vi "Test UI-Bus Boolean Vars.vi"() -> ()   [LabVIEW 2021]
uses:
  Source/UI-Bus/UI-Bus.lvclass
  C:/Program Files (x86)/National Instruments/LabVIEW 2021/vi.lib/TSA/Omni-Bus/Omni-Bus/Bus Access/Bus_Access.lvclass
  <vilib>/TSA/Omni-Bus/Omni-Bus/Omni_Bus.lvclass
  <vilib>/TSA/Omni-Bus/Omni-Bus/Support/Broad Types.ctl
  <vilib>/TSA/Abstract Data Classes/Abs_Types/Type/Abs_Type.lvclass/Abs_Type.ctl
  <vilib>/TSA/Omni-Bus/Omni-Bus/Omni_Bus.lvclass/Omni_Bus.ctl
  <vilib>/TSA/Omni-Bus/Omni-Bus/Support/Read/Read Multi Boolean.vi
  <vilib>/TSA/Omni-Bus/Omni-Bus/Support/Write/Write Boolean.vi
  <vilib>/TSA/Omni-Bus/Omni-Bus/Support/Get/Get Multi Boolean.vi
  <vilib>/TSA/Omni-Bus/Omni-Bus/Support/FindVar.vi
  <vilib>/TSA/Omni-Bus/Omni-Bus/Support/FindMultiVar.vi
  <vilib>/Utility/error.llb/Clear Errors.vi
  <vilib>/TSA/Omni-Bus/Omni-Bus/Properties/Read Var Map.vi
  <vilib>/TSA/Abstract Data Classes/Abs_Types/Type/Properties/Read Tag.vi
  <vilib>/TSA/Abstract Data Classes/Abs_Types/Boolean/Abs_Boolean.lvclass
  C:/Program Files (x86)/National Instruments/LabVIEW 2021/vi.lib/TSA/Abstract Data Classes/Abs_Types/Type/Abs_Type.lvclass
  <vilib>/TSA/Abstract Data Classes/Abs_Types/Value/Abs_Value.lvclass
  <vilib>/TSA/Omni-Bus/Omni-Bus/Support/Check For Read Only Error.vi
  <vilib>/TSA/Omni-Bus/Omni-Bus/Support/Incorrect Tag String Error.vi
  <vilib>/TSA/Abstract Data Classes/Abs_Types/Type/Abs_Type.lvclass
panel:
  in  "Tag List":string(combo)
  out "Boolean 8":bool
  in  "OK Button 5":bool
  in  "OK Button 4":bool
  in  "OK Button 3":bool
  in  "OK Button 2":bool
  in  "OK Button":bool
  in  "Boolean 7":bool
  in  "Boolean 6":bool
  in  "Boolean 5":bool
  out "error":errorcluster
  in  "stop":bool
  out "Booleans":bool[](array[boolean])
  out "Tags":string[](array[string])
  out "Boolean 4":bool
  out "Boolean 3":bool
  in  "Boolean 2":bool
  in  "Boolean":bool
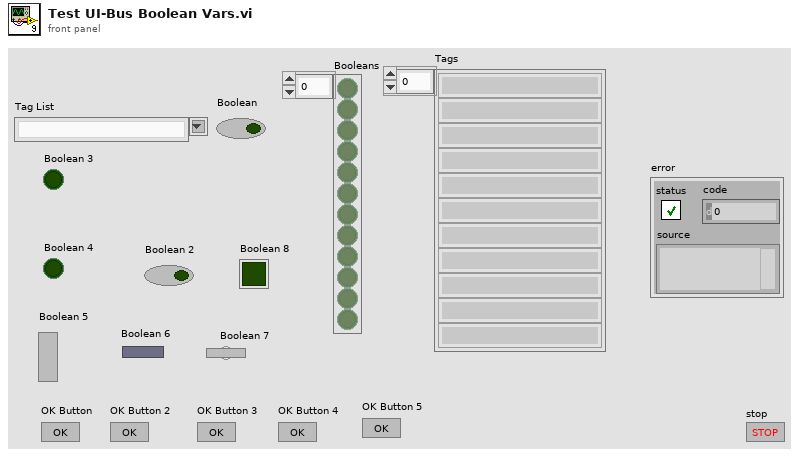
[diagram p1: front panel]
types:
  T1 = typedef "Omni_Bus.lvclass/Broad Types.ctl" = enum16{"All Tags", "NI Specific Type", "Boolean", "String", "Numeric", "Float", "Integer", "Collection", "All Value Types", "Non Value Types"}
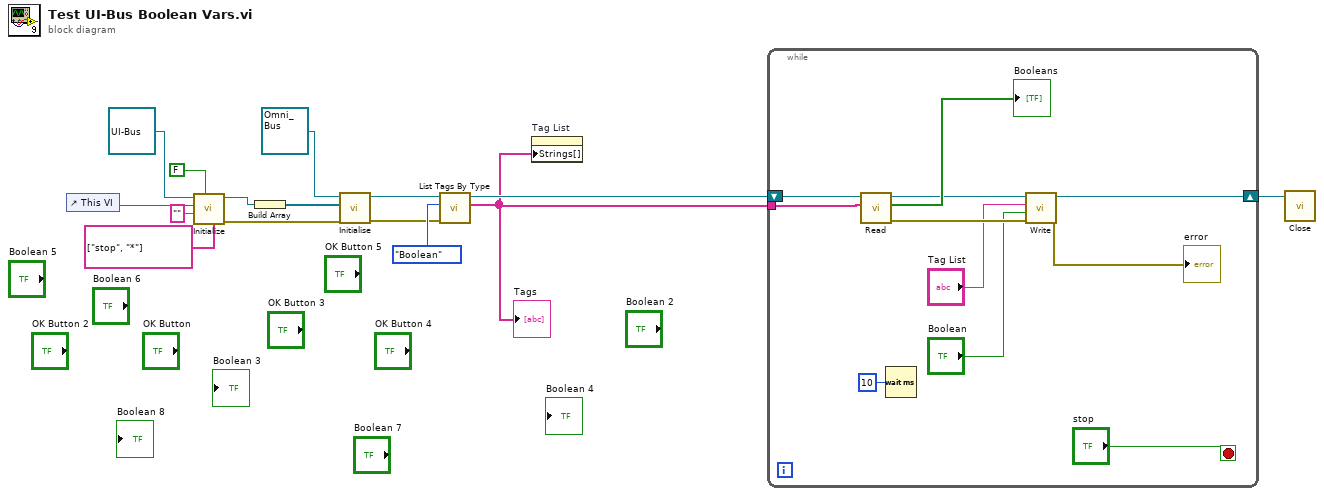
[diagram p0: block diagram]
diagram:
  n1 = control-ref of="This VI"() -> (w14:refnum<vi>)
  n2 = call "Initialize.vi"("Label Black List"=string[] ["stop", "*"], "Tab Label in Tag"=FALSE, "Tag Root"="", "VI Refnum"=w14, "UI-Bus in"=refnum<class "UI-Bus.lvclass"> refnum) -> ("error out"=w10:errorcluster, "UI-Bus out"=w12:refnum<class "UI-Bus.lvclass">)  [unwired: 5 in]
  n3 = Build Array(w12) -> (w11:refnum<class "UI-Bus.lvclass">[])
  n4 = call-dynamic "Initialise.vi"("error in (no error)"=w10, "Bus Access"=w11, "Var Bus in"=refnum<class "Omni_Bus.lvclass"> refnum) -> ("error out"=w2:errorcluster, "Var Bus out"=w3:refnum<class "Omni_Bus.lvclass">)  [unwired: 7 in]
  n5 = call <vilib>:"List Tags By Type.vi"("error in (no error)"=w2, "Broad Types"=Broad_Types."Boolean", "Var Bus in"=w3) -> ("Tags"=w1:string[], "Var Bus out"=w8:refnum<class "Omni_Bus.lvclass">)  [unwired: 5 in, 2 out]
  "Tags" <- w1
  n6 = property on="Tag List" class="CmbBox"("Strings[]"=w1) -> ()  [unwired: 2 in, 2 out]
  n7 = while {
    tunnel: w1 -> [w26]
    shift-right: [w19] -> w7
    shift-left: w8 -> [w25]
    stop <- "stop" stop-if-true
    n8 = call-poly <vilib>:"Read.vi"("Tags"=w26, "Var Bus in"=w25) -> ("error out"=w20:errorcluster, "Booleans"=→"Booleans":bool[], "Var Bus out"=w21:refnum<class "Omni_Bus.lvclass">)  [unwired: 7 in]
    n9 = Wait (ms)(milliseconds to wait=u32 10) -> ()  [unwired: 1 out]
    n10 = call-poly <vilib>:"Write.vi"("error in (no error)"=w20, "Boolean"="Boolean", "Tag"="Tag List", "Omni_Bus in"=w21) -> ("error out"=→"error":errorcluster, "Omni_Bus out"=w19:refnum<class "Omni_Bus.lvclass">)  [unwired: 6 in]
  }
  n11 = call-dynamic "Close.vi"("Data in"=w7) -> ()  [unwired: 9 in, 2 out]
